vi "Send Data.vi"(8 "error in (no error)":errorcluster, 11 "RT - Analysis Data in in":T1 {"Cutoff Frequncies"."HP Passband" min=1.0 step=1.0 format="%#.4f"; "Cutoff Frequncies"."LP Stopband" min=1.0 step=1.0 format="%#.4f"; "Cutoff Frequncies"."HP Stopband" min=1.0 step=1.0 format="%#.4f"; "Cutoff Frequncies"."LP Passband" min=1.0 step=1.0 format="%#.4f"}) -> (0 "error out":errorcluster, 3 "RT - Analysis Data out":T1 {"Cutoff Frequncies"."HP Passband" min=1.0 step=1.0 format="%#.4f"; "Cutoff Frequncies"."LP Stopband" min=1.0 step=1.0 format="%#.4f"; "Cutoff Frequncies"."HP Stopband" min=1.0 step=1.0 format="%#.4f"; "Cutoff Frequncies"."LP Passband" min=1.0 step=1.0 format="%#.4f"})   [LabVIEW 2018]
doc: "If the earliest data point in the array of data is older than half of the Front Panel update rate, send data and clear array."
uses:
  Variables/Global - cRIO Configuration Options.vi
  Top Level/Shared Controls/cRIO State.ctl
  Top Level/Shared Controls/Analyzed Data Sets.ctl
  Top Level/Shared Controls/All Data Cluster.ctl
  Top Level/Shared Controls/Acq Data.ctl
  Top Level/Shared Controls/Post-Analysis Data.ctl
  Top Level/Shared Controls/Calculated Data.ctl
  Private Controls/RT-Analysis Data.ctl
  RT - Analysis.lvlib
  Top Level/Shared Controls/Parsed Tag Cluster.ctl
  Private Controls/Parsed Data Arrays.ctl
  Modules/Testing UI 3/Private Controls/Cutoff Frequency.ctl
  Modules/Testing UI 3/Testing UI 3.lvlib
  Top Level/Shared Controls/APU Setup File.ctl
panel:
  # "Highpass Cutoff Frequency"
  # "Lowpass Cutoff Frequency"
  # "Highpass Cutoff Frequency"
  # "Lowpass Cutoff Frequency"
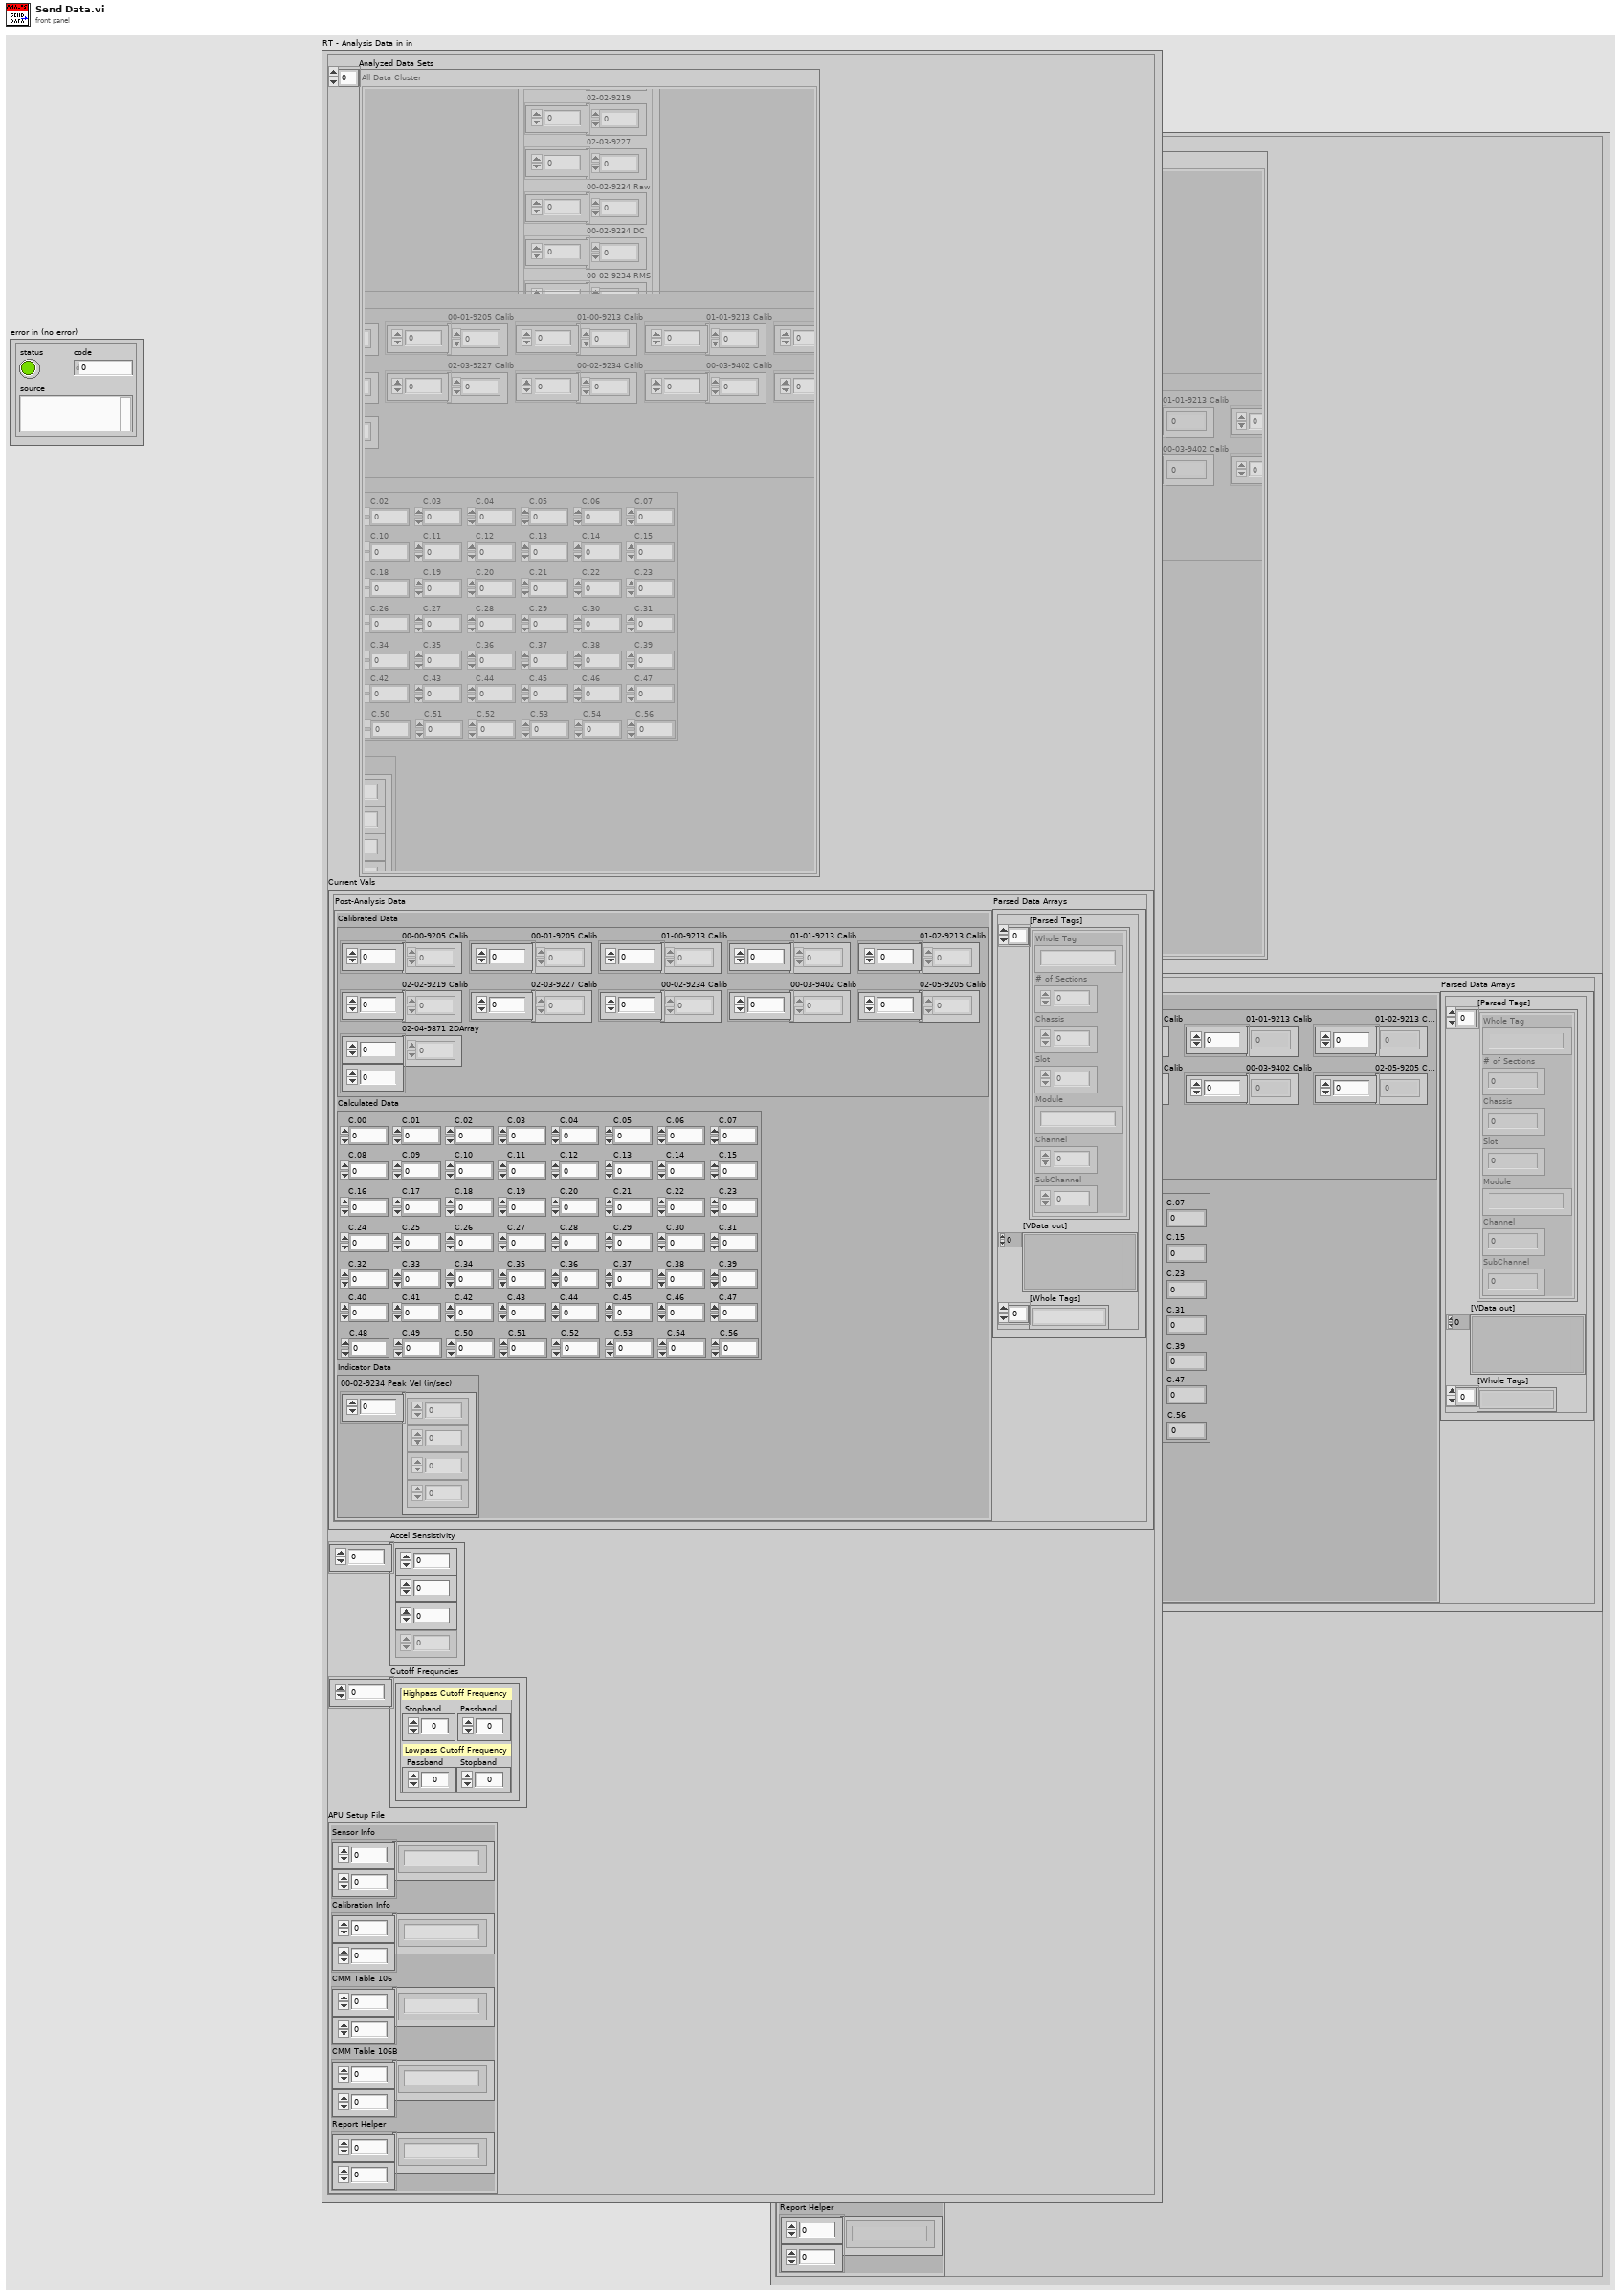
[diagram p1: front panel]
types:
  T1 = typedef "RT - Analysis.lvlib/RT-Analysis Data.ctl" = cluster{"Analyzed Data Sets":T2, "Current Vals":cluster{"Post-Analysis Data":T5, "Parsed Data Arrays":T7}, "Accel Sensistivity":dbl[], "Cutoff Frequncies":T9[], "APU Setup File":T10}
  T2 = typedef "Analyzed Data Sets.ctl" = T3[]
  T3 = typedef "All Data Cluster.ctl" = cluster{"Acq Data":T4, "Post-Analysis Data":T5}
  T4 = typedef "Acq Data.ctl" = cluster{"00-00-9220":dbl[], "00-01-9220":dbl[], "01-00-9213":dbl[], "01-01-9213":dbl[], "01-02-9213":dbl[], "02-02-9219":dbl[], "02-03-9227":dbl[], "00-02-9234 Raw":dbl[], "00-02-9234 DC":dbl[], "00-02-9234 RMS":dbl[], "00-02-9234 Peak":dbl[], "00-02-9234 Freq":dbl[], "00-03-9402":dbl[], "02-05-9205":dbl[], "02-04-9871":dbl[], "Timestamp":timestamp}
  T5 = typedef "Post-Analysis Data.ctl" = cluster{"Calibrated Data":cluster{"00-00-9205 Calib":dbl[], "00-01-9205 Calib":dbl[], "01-00-9213 Calib":dbl[], "01-01-9213 Calib":dbl[], "01-02-9213 Calib":dbl[], "02-02-9219 Calib":dbl[], "02-03-9227 Calib":dbl[], "00-02-9234 Calib":dbl[], "00-03-9402 Calib":dbl[], "02-05-9205 Calib":dbl[], "02-04-9871 2DArray":dbl[][]}, "Calculated Data":T6, "Indicator Data":cluster{"00-02-9234 Peak Vel (in/sec)":dbl[]}}
  T6 = typedef "Calculated Data.ctl" = cluster{"C.00":dbl, "C.01":dbl, "C.02":dbl, "C.03":dbl, "C.04":dbl, "C.05":dbl, "C.06":dbl, "C.07":dbl, "C.08":dbl, "C.09":dbl, "C.10":dbl, "C.11":dbl, "C.12":dbl, "C.13":dbl, "C.14":dbl, "C.15":dbl, "C.16":dbl, "C.17":dbl, "C.18":dbl, "C.19":dbl, "C.20":dbl, "C.21":dbl, "C.22":dbl, "C.23":dbl, "C.24":dbl, "C.25":dbl, "C.26":dbl, "C.27":dbl, "C.28":dbl, "C.29":dbl, "C.30":dbl, "C.31":dbl, "C.32":dbl, "C.33":dbl, "C.34":dbl, "C.35":dbl, "C.36":dbl, "C.37":dbl, "C.38":dbl, "C.39":dbl, "C.40":dbl, "C.41":dbl, "C.42":dbl, "C.43":dbl, "C.44":dbl, "C.45":dbl, "C.46":dbl, "C.47":dbl, "C.48":dbl, "C.49":dbl, "C.50":dbl, "C.51":dbl, "C.52":dbl, "C.53":dbl, "C.54":dbl, "C.56":dbl}
  T7 = typedef "RT - Analysis.lvlib/Parsed Data Arrays.ctl" = cluster{"[Parsed Tags]":T8[], "[VData out]":variant[], "[Whole Tags]":string[]}
  T8 = typedef "Parsed Tag Cluster.ctl" = cluster{"Whole Tag":string, "# of Sections":u8, "Chassis":u8, "Slot":u8, "Module":string, "Channel":u8, "SubChannel":u8}
  T9 = typedef "Testing UI 3.lvlib/Cutoff Frequency.ctl" = cluster{"LP Passband":dbl, "HP Stopband":dbl, "LP Stopband":dbl, "HP Passband":dbl}
  T10 = typedef "APU Setup File.ctl" = cluster{"Sensor Info":string[][], "Calibration Info":string[][], "CMM Table 106":string[][], "CMM Table 106B ":string[][], "Report Helper":string[][]}
  T11 = typedef "cRIO State.ctl" = enum16{"Waiting for Cal Info", "Idle", "Calibration", "Testing"}
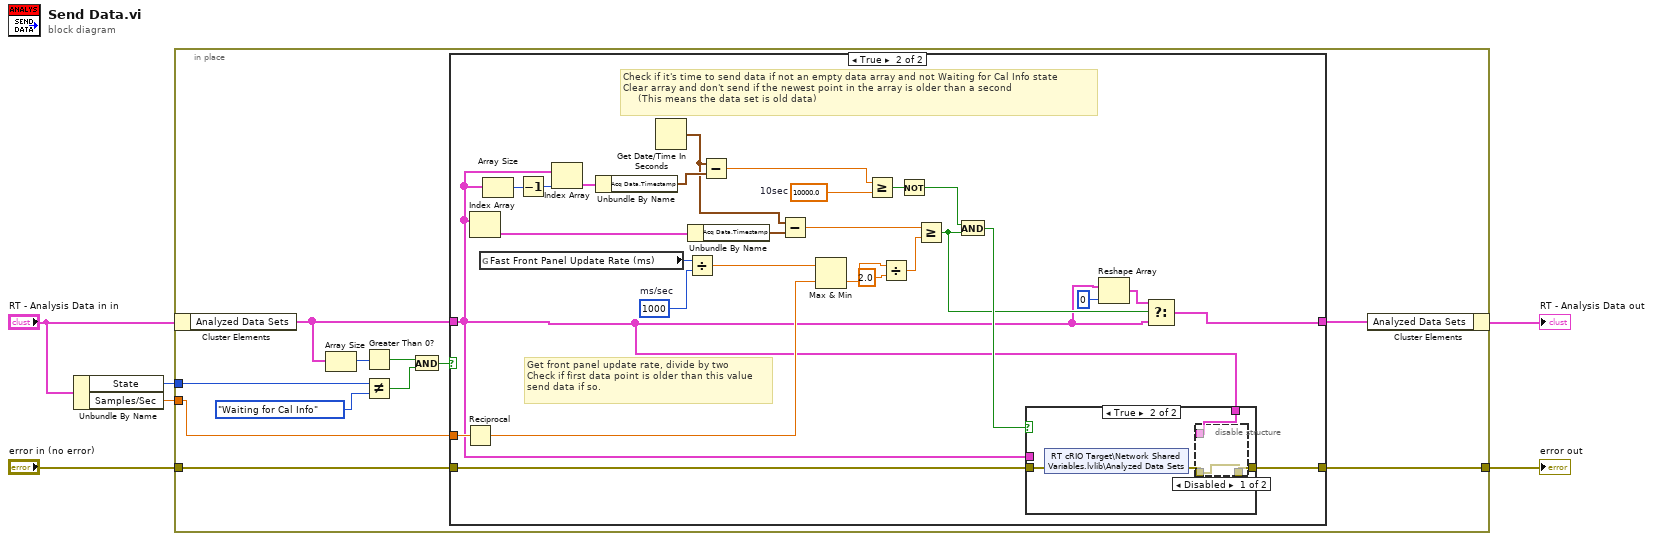
[diagram p0: block diagram]
diagram:
  n1 = Unbundle By Name("RT - Analysis Data in in") -> ("State"=w2:T11, "Samples/Sec"=w1:dbl)
  n2 = in-place {
    in-place-border: "error in (no error)" -> [w16]
    in-place-border: [w15] -> w6
    in-place-border: w2 -> [w9]
    in-place-border: w1 -> [w7]
    n3 = in-place-cluster #1("RT - Analysis Data in in") -> ("Analyzed Data Sets"=w13:T2)
    n4 = Array Size(array=w13) -> (size(s)=w14:i32)
    n5 = Greater Than 0?(x=w14) -> (x > 0?=w11:bool)
    n6 = Not Equal?(x=w9, y=cRIO_State."Waiting for Cal Info") -> (x != y?=w10:bool)
    n7 = And(x=w11, y=w10) -> (x .and. y?=w12:bool)
    n8 = case shown="True" w12 {
      tunnel: [w19 w42] -> w17
      tunnel: w16 -> [w18 w41]
      tunnel: [w18 w40] -> w15
      tunnel: w13 -> [w19 w20]
      tunnel: w7 -> [_ w26]
      frame False {
      }
      frame True {
        w36 = 10000.0  # 10sec
        w44 = 1000  # ms/sec
        # "Check if it's time to send data if not an empty data array and not Waiting for Cal Info state\nClear array and don't send if the newest point in the array is older than a second\n     (This means the data set is old data)"
        # "Get front panel update rate, divide by two\nCheck if first data point is older than this value\nsend data if so."
        n9 = Reciprocal(x=w26) -> (1/x=w24:dbl)
        n10 = Index Array(array=w20) -> (element=w47:T3)  [unwired: 1 in]
        n11 = global read "Global - cRIO Configuration Options.vi" "Fast Front Panel Update Rate (ms)"() -> (w45:i32)
        n12 = Array Size(array=w20) -> (size(s)=w32:i32)
        n13 = Decrement(x=w32) -> (x-1=w31:i32)
        n14 = Index Array(array=w20, index=w31) -> (element=w30:T3)
        n15 = Unbundle By Name(w30) -> ("Acq Data.Timestamp"=w29:timestamp)
        n16 = Get Date/Time In Seconds() -> (seconds since 1Jan1904=w22:timestamp)
        n17 = Divide(x=w45, y=w44) -> (x/y=w23:dbl)
        n18 = Unbundle By Name(w47) -> ("Acq Data.Timestamp"=w46:timestamp)
        n19 = Subtract(x=w22, y=w29) -> (x-y=w28:dbl)
        n20 = Subtract(x=w22, y=w46) -> (x-y=w37:dbl)
        n21 = Max & Min(x=w23, y=w24) -> (min(x,y)=w25:dbl)  [unwired: 1 out]
        n22 = Greater Or Equal?(x=w28, y=w36) -> (x >= y?=w34:bool)
        n23 = Divide(x=w25, y=2.0) -> (x/y=w21:dbl)
        n24 = Not(x=w34) -> (.not. x?=w33:bool)
        n25 = Greater Or Equal?(x=w37, y=w21) -> (x >= y?=w27:bool)
        n26 = And(x=w33, y=w27) -> (x .and. y?=w35:bool)
        n27 = case shown="True" w35 {
          tunnel: w41 -> [w48 w52]
          tunnel: [w48 w50] -> w40
          tunnel: w20 -> [_ _]
          tunnel: w20 -> [_ w49]
          frame False {
          }
          frame True {
            n28 = shared-variable "RT cRIO Target\\Network Shared Variables.lvlib\\Analyzed Data Sets"(error in=w52) -> (error out=w51:errorcluster)  [unwired: 1 in]
            n29 = disable-structure shown="Disabled" {
              disable-tunnel: w51 -> [w53 w54]
              disable-tunnel: [w53 w54] -> w50
              disable-tunnel: w49 -> [_ _]
              frame Disabled {
              }
              frame Enabled {
              }
            }
          }
        }
        n30 = Reshape Array(w20, 0 ("dimension size")) -> (w38:T2)
        n31 = Select(t=w38, s=w27, f=w20) -> (s? t:f=w42:T2)
      }
    }
    n32 = in-place-cluster #1("Analyzed Data Sets"=w17) -> (→"RT - Analysis Data out":T1)
  }
  "error out" <- w6
